vi "data save in xcel.vi"(6 "Data":string[][](array[string]), 7 "Condition":bool, 10 "Report Type":string, 11 "Temp Path":path) -> (0 "error out":errorcluster)   [LabVIEW 2024]
uses:
  <vilib>/Utility/NIReport.llb/Append Text Table to Report (wrap).vi
  <vilib>/Utility/NIReport.llb/NI_report.lvclass
panel:
  out "array w/ subset deleted":string[][](array[string])
  out "Column Header Strings[]":string[](array[string])=["No.", "Date & Time", "Model Name", "Part No.", "Sr. No.", "Oilways Leak Value(ml/min)", "Oilways Leak Result", "Waterways Leak\nValue(ml/min)", "Waterways Leak Result", "Resutl"]
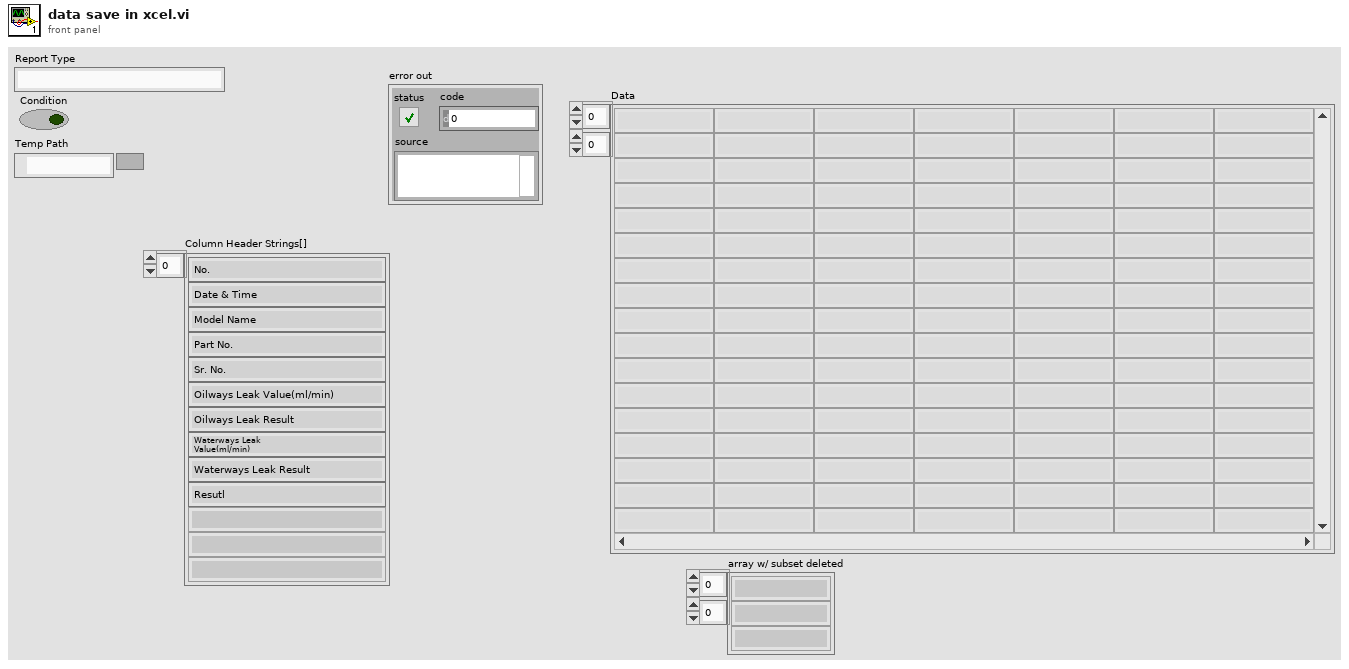
[diagram p1: front panel]
types:
  T1 = enum16{"maximized", "minimized", "normal", "no change"}
  T2 = enum16{"Standard Report", "HTML", "Word", "Excel"}
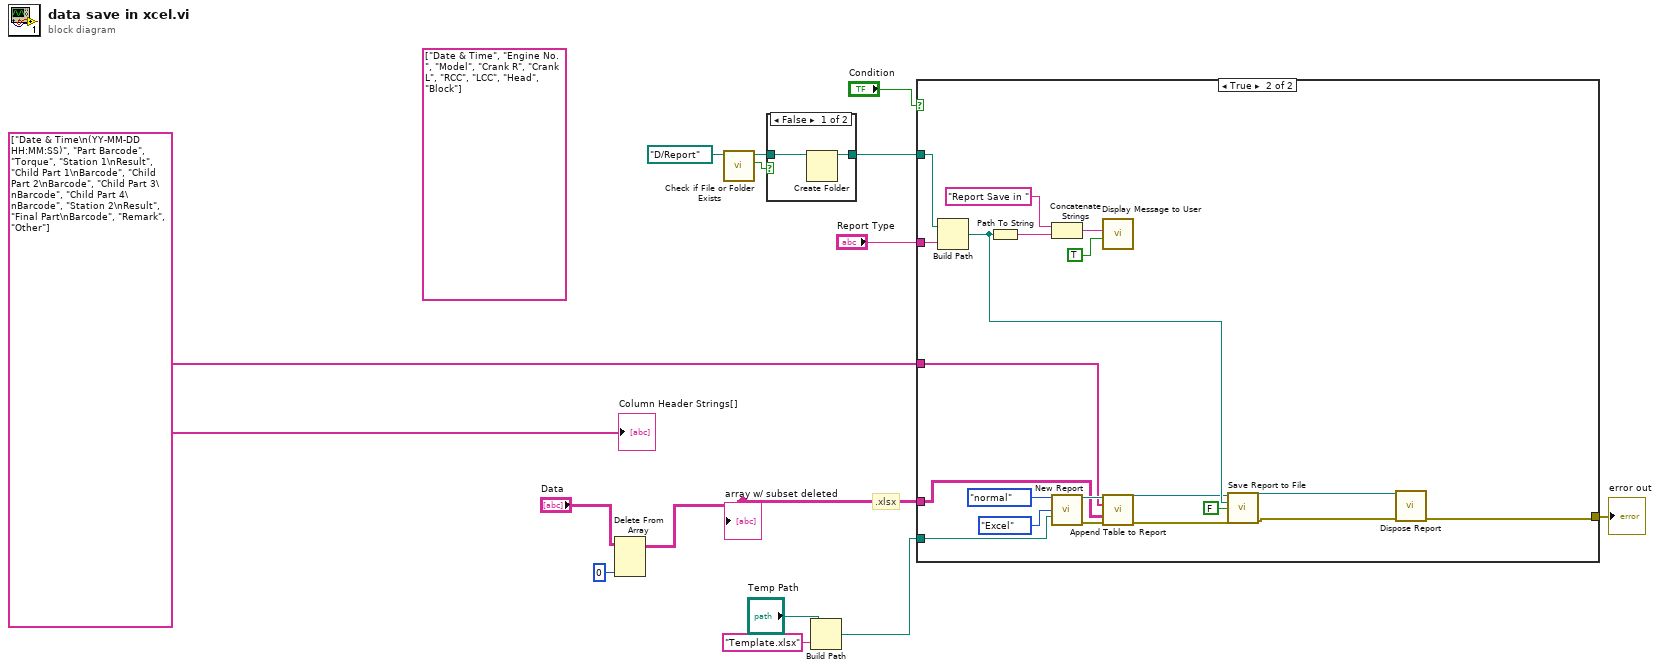
[diagram p0: block diagram]
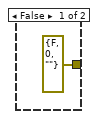
[diagram p3: hidden frame]
diagram:
  w1 = string[] ["Date & Time\n(YY-MM-DD HH:MM:SS)", "Part Barcode", "Torque", "Station 1\nResult", "Child Part 1\nBarcode", "Child Part 2\nBarcode", "Child Part 3\nBarcode", "Child Part 4\nBarcode", "Station 2\nResult", "Final Part\nBarcode", "Remark", "Other"] ("Column Header Strings[]")
  (unwired) string[] ["Date & Time", "Engine No.", "Model", "Crank R", "Crank L", "RCC", "LCC", "Head", "Block"] ("Column Header Strings[]")
  # ".xlsx"
  n1 = Delete From Array(array="Data", index (col)=0 ("disabled index (col)")) -> (array with subset deleted=w3:string[][])  [unwired: 2 in, 1 out]
  "array w/ subset deleted" <- w3
  n2 = call <vilib>:"Check if File or Folder Exists.vi"("path"=path "D:/Report" ("selected path 2")) -> ("file or folder exists?"=w11:bool, "dup path"=w10:path)  [unwired: 8 in, 1 out]
  n3 = case shown="False" w11 {
    tunnel: w10 -> [w16 w17]
    tunnel: [w15 w17] -> w9
    frame False {
      n4 = Create Folder(path (use dialog)=w16) -> (created path=w15:path)  [unwired: 2 in, 2 out]
    }
    frame True {
    }
  }
  n5 = Build Path(base path="Temp Path", name or relative path="Template.xlsx") -> (appended path=w5:path)
  n6 = case shown="True" "Condition" {
    tunnel: w9 -> [_ w38]
    tunnel: "Report Type" -> [_ w37]
    tunnel: w3 -> [_ w26]
    tunnel: w1 -> [_ w27]
    tunnel: w5 -> [_ w30]
    tunnel: [errorcluster {"status"=FALSE, "code"=0, "source"=""} ("error out") w19] -> w8
    frame False {
    }
    frame True {
      n7 = Build Path(base path=w38, name or relative path=w37) -> (appended path=w21:path)
      n8 = Path To String(path=w21) -> (string=w34:string)
      n9 = Concatenate Strings("Report Save in " ("string"), w34) -> (w33:string)
      n10 = call <vilib>:"New Report.vi"("window state (normal)"=T1."normal", "report type"=T2."Excel", "template (empty)"=w30) -> ("report out"=w29:refnum<class "NI_report.lvclass">, "error out"=w28:errorcluster)  [unwired: 11 in]
      n11 = call "Display Message to User"("Enable"=TRUE, "Message"=w33) -> ()  [unwired: 8 in, 2 out]
      n12 = call-poly <vilib>:"Append Table to Report.vi"("report in"=w29, "column headers"=w27, "text data"=w26, "error in (no error)"=w28) -> ("report out"=w20:refnum<class "NI_report.lvclass">, "error out"=w22:errorcluster)  [unwired: 8 in, 2 out]
      n13 = call-dynamic "Save Report to File.vi"("report in"=w20, "report file path"=w21, "prompt to replace? (F)"=FALSE, "error in (no error)"=w22) -> ("report out"=w25:refnum<class "NI_report.lvclass">, "error out"=w24:errorcluster)  [unwired: 10 in]
      n14 = call-dynamic "Dispose Report.vi"("report in"=w25, "error in (no error)"=w24) -> ("error out"=w19:errorcluster)  [unwired: 13 in]
    }
  }
  "error out" <- w8
  "Column Header Strings[]" <- w1
